vi "Vector3DYaw.vi"(0 "Vector3D":T1, 3 "Theta":dbl) -> (7 "Rotated Vector3D":T1)   [LabVIEW 2018]
uses:
  Vector3D.ctl
  Vector3DtoVector2D_XY.vi
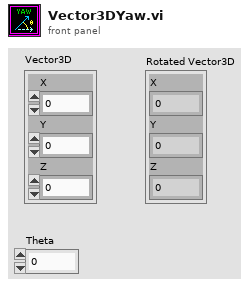
[diagram p1: front panel]
types:
  T1 = typedef "Vector3D.ctl" = cluster{"X":dbl, "Y":dbl, "Z":dbl}
  T2 = typedef "Vector2D.ctl" = cluster{"X":dbl, "Y":dbl}
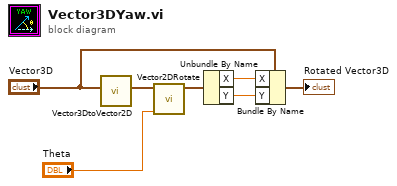
[diagram p0: block diagram]
diagram:
  n1 = call-poly "Vector3DtoVector2D.vi"("Vector3D"="Vector3D") -> ("Vector2D"=w5:T2)  [unwired: 10 in]
  n2 = call "Vector2DRotate.vi"("Vector"=w5, "Theta"="Theta") -> ("Rotated Vector"=w3:T2)  [unwired: 8 in]
  n3 = Unbundle By Name(w3) -> ("X"=w2:dbl, "Y"=w1:dbl)
  n4 = Bundle By Name(cluster="Vector3D", "X"=w2, "Y"=w1) -> (→"Rotated Vector3D":T1)
